vi "溶解氧校准.vi"(8 "error in (no error)":errorcluster caption="错误输入（无错误）", 9 "标液二":cluster{"信号值":sgl}, 10 "标液一":cluster{"信号值":sgl}, 11 "校准方式":enum16{"单点校准", "两点校准"}(ring)) -> (0 "error out":errorcluster caption="错误输出")   [LabVIEW 2016, in "NAQ_DO.lvlib"]
uses:
  NAQ_DO.lvlib
  <vilib>/Plasmionique/MB Master/MB_Master/MB_Master.lvclass
  <vilib>/Plasmionique/MB Master/MB Master.lvlib
  elevator/elevator.lvlib
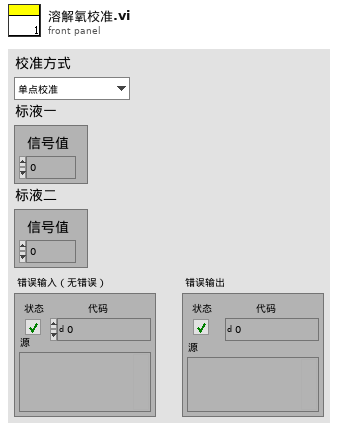
[diagram p1: front panel]
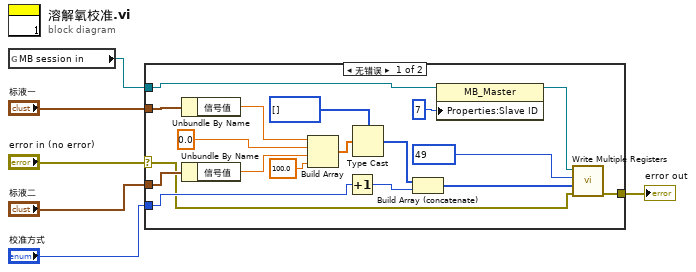
[diagram p0: block diagram]
diagram:
  n1 = global read "elevator 全局变量.vi" "MB session in"() -> (w1:refnum<class "MB_Master.lvclass">)
  n2 = case shown="无错误" "error in (no error)" {
    selector: "error in (no error)" -> [w10 w25]
    tunnel: [w24 w25] -> w6
    tunnel: "标液一" -> [w23 _]
    tunnel: "标液二" -> [w22 _]
    tunnel: "校准方式" -> [w19 _]
    tunnel: w1 -> [w7 _]
    frame No Error {
      n3 = Unbundle By Name(w23) -> ("信号值"=w21:sgl)
      n4 = Unbundle By Name(w22) -> ("信号值"=w20:sgl)
      n5 = Build Array(w21, sgl 0.0 ("信号值"), w20, sgl 100.0 ("信号值")) -> (w12:sgl[])
      n6 = Increment(x=w19) -> (x+1=w18:enum16{"单点校准", "两点校准"})
      n7 = Type Cast(type=u16[] [], x=w12) -> (*(type *) &x=w11:u16[])
      n8 = Build Array (concatenate)(w11, w18) -> (w14:u16[])
      n9 = property class="MB_Master"(reference=w7, "Properties:Slave ID"=7) -> (reference out=w16:refnum<class "MB_Master.lvclass">)  [unwired: 1 in, 1 out]
      n10 = call <vilib>:"Write Multiple Registers.vi"("error in (no error)"=w10, "values"=w14, "starting address"=u16 49, "MB session in"=w16) -> ("error out"=w24:errorcluster)  [unwired: 6 in, 1 out]
    }
    frame Error {
    }
  }
  "error out" <- w6
